vi "AvgByGroups.vi"() -> ()   [LabVIEW 2016]
panel:
  out "Array":dbl[](array[numeric])
  out "output array":dbl[][](array[numeric])
  out "size(s) 2":i32
  out "subarray":dbl[](array[numeric])
  out "x-y*floor(x/y)":dbl
  out "floor(x/y)":dbl
  out "size(s)":i32
  in  "Groups2Avg":dbl
  out "Y":dbl[](array[numeric])
  out "X":dbl[](array[numeric])
  in  "Stops (averaged) vs time":cluster{dbl[], dbl[]}(graph)
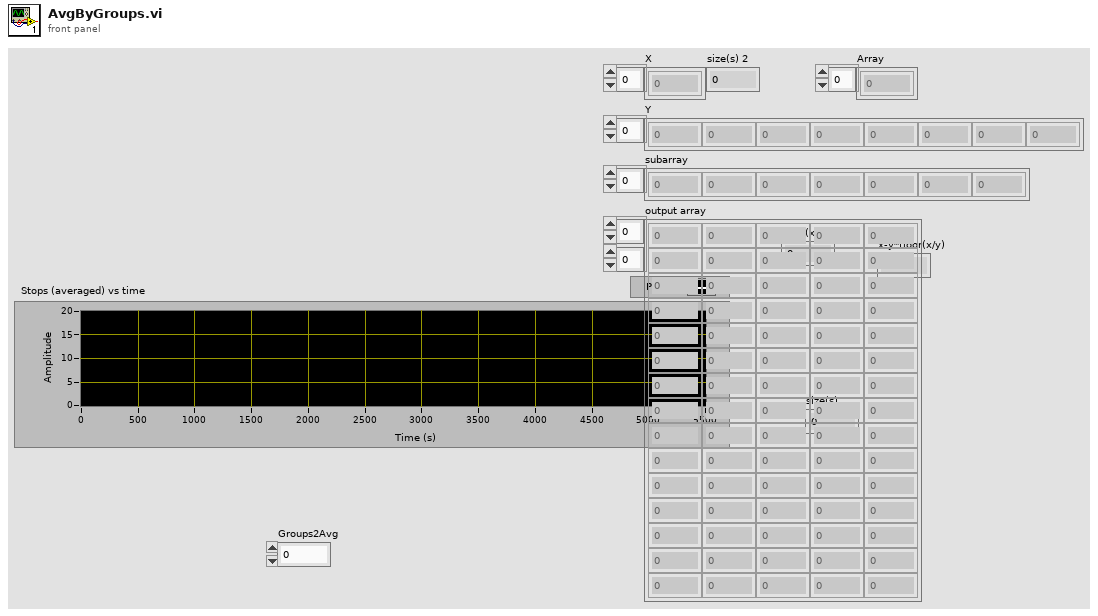
[diagram p1: front panel]
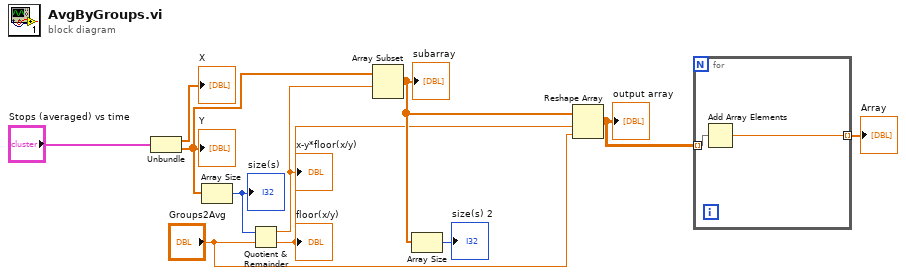
[diagram p0: block diagram]
diagram:
  n1 = Unbundle("Stops (averaged) vs time") -> (→"X":dbl[], w7:dbl[])
  "Y" <- w7
  n2 = Array Size(array=w7) -> (size(s)=w9:i32)
  "size(s)" <- w9
  n3 = Quotient & Remainder(x=w9, y="Groups2Avg") -> (x-y*floor(x/y)=w8:dbl, floor(x/y)=w4:dbl)
  "floor(x/y)" <- w4
  "x-y*floor(x/y)" <- w8
  n4 = Array Subset(array=w7, index=w8) -> (w5:dbl[])  [unwired: 1 in]
  "subarray" <- w5
  n5 = Array Size(array=w5) -> (size(s)=→"size(s) 2":i32)
  n6 = Reshape Array(w5, w4, "Groups2Avg") -> (w2:dbl[][])
  "output array" <- w2
  n7 = for {
    tunnel: w2 -> [w13] mode=indexing
    tunnel: [w12] -> w1 mode=indexing
    n8 = Add Array Elements(numeric array=w13) -> (sum=w12:dbl)
  }
  "Array" <- w1
